vi "OscConnect-Com-Exec.vi"(8 "error in (no error)":errorcluster, 9 "ControlQueue":refnum<queue>, 10 "data":variant, 11 "Oscilloscope in":refnum<class "Oscilloscope.lvclass">) -> (0 "error out":errorcluster, 3 "Oscilloscope out":refnum<class "Oscilloscope.lvclass">)   [LabVIEW 2015, in "Oscilloscope.lvclass"]
uses:
  Oscilloscope.lvclass
  dependecies/ControlsVIs/Clusters-def/SERVER-Commands.ctl
  dependecies/ControlsVIs/Clusters-def/OSc-Reply-to-Connect.ctl
  dependecies/ControlsVIs/Clusters-def/OSc-Reply-Connect-client.ctl
  GeneralFunctionality/GeneralFunctionality.lvclass/GeneralFunctionality.ctl
  Control/Control-Server/Control-Server.lvclass
  GeneralFunctionality/GeneralFunctionality.lvclass
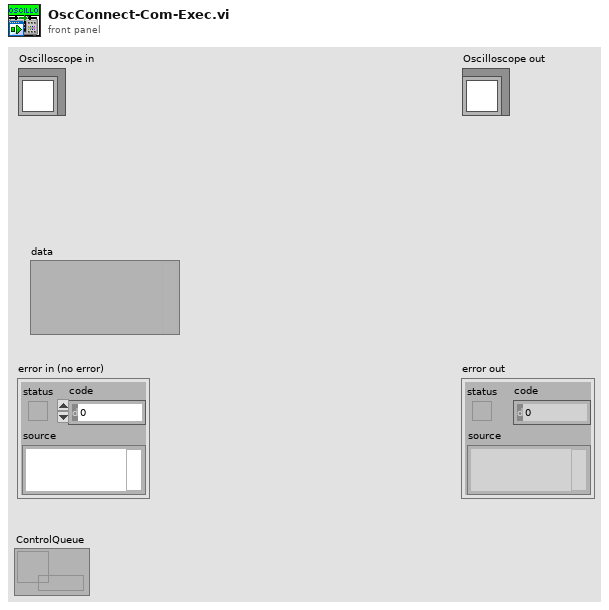
[diagram p1: front panel]
types:
  T1 = typedef "Control-Server.lvclass/SERVER-Commands.ctl" = string
  T2 = typedef "Oscilloscope.lvclass/OSc-Reply-Connect-Client.ctl" = cluster{"on/off":bool, "WCM_state":bool, "error":errorcluster}
  T3 = typedef "Oscilloscope.lvclass/OSc-Reply-to-Connect.ctl" = cluster{"On/Off":bool, "error":errorcluster, "Oscilloscope.lvclass":refnum<class "Oscilloscope.lvclass">}
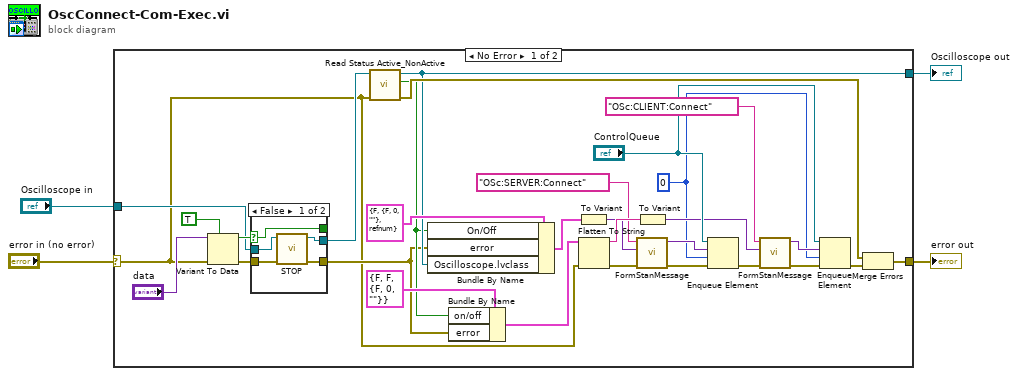
[diagram p0: block diagram]
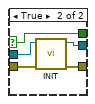
[diagram p2: hidden frame]
diagram:
  n1 = case shown="No Error" "error in (no error)" {
    selector: "error in (no error)" -> [w18 w46]
    tunnel: [w27 w46] -> w3
    tunnel: [w25 w45] -> w1
    tunnel: "Oscilloscope in" -> [w30 w45]
    frame No Error {
      w5 = 0 ("timeout en ms (-1)")
      n2 = Variant To Data(error in=w18, type=TRUE, Variant="data") -> (data=w32:bool, error out=w31:errorcluster)
      n3 = case shown="False" w32 {
        selector: w32 -> [w35 w40]
        tunnel: w31 -> [w39 w44]
        tunnel: w30 -> [w37 w43]
        tunnel: [w36 w42] -> w24
        tunnel: [w38 w41] -> w21
        tunnel: [w35 w40] -> _
        frame False {
          n4 = call-dynamic "STOP.vi"("error in (no error)"=w39, "Stop in"=w37) -> ("error out"=w38:errorcluster, "Stop out"=w36:refnum<class "Oscilloscope.lvclass">)  [unwired: 8 in]
        }
        frame True {
          n5 = call-dynamic "INIT.vi"("error in (no error)"=w44, "GeneralFunctionality in"=w43) -> ("error out"=w41:errorcluster, "GeneralFunctionality out"=w42:refnum<class "Oscilloscope.lvclass">)  [unwired: 8 in]
        }
      }
      n6 = call "Read Status Active_NonActive.vi"("error in (no error)"=w18, "GeneralFunctionality in"=w24) -> ("error out"=w28:errorcluster, "Status Active/NonActive"=w22:bool, "GeneralFunctionality out"=w25:refnum<class "Oscilloscope.lvclass">)  [unwired: 7 in]
      n7 = Bundle By Name(cluster=T3 {"On/Off"=FALSE, "error"={"status"=FALSE, "code"=0, "source"=""}, "Oscilloscope.lvclass"=refnum} ("Cluster"), "On/Off"=w22, "error"=w21, "Oscilloscope.lvclass"=w25) -> (w29:T3)
      n8 = Bundle By Name(cluster=T2 {"on/off"=FALSE, "WCM_state"=FALSE, "error"={"status"=FALSE, "code"=0, "source"=""}} ("output cluster"), "on/off"=w22, "error"=w21) -> (w20:T2)
      n9 = To Variant(anything=w29) -> (Variant=w8:variant)
      n10 = Flatten To String(anything=w20, error in (no error)=w18) -> (data string=w19:string, error out=w16:errorcluster)  [unwired: 2 in, 1 out]
      n11 = call "FormStanMessage.vi"("error in"=w16, "data"=w8, "Command"=T1 "OSc:SERVER:Connect" ("Commands")) -> ("error out"=w15:errorcluster, "message"=w14:variant)  [unwired: 7 in]
      n12 = To Variant(anything=w19) -> (Variant=w6:variant)
      n13 = Enqueue Element(queue="ControlQueue", element=w14, timeout in ms (-1)=w5, error in (no error)=w15) -> (error out=w13:errorcluster)  [unwired: 2 out]
      n14 = call "FormStanMessage.vi"("error in"=w13, "data"=w6, "Command"=T1 "OSc:CLIENT:Connect" ("Commands")) -> ("error out"=w12:errorcluster, "message"=w7:variant)  [unwired: 7 in]
      n15 = Enqueue Element(queue="ControlQueue", element=w7, timeout in ms (-1)=w5, error in (no error)=w12) -> (error out=w11:errorcluster)  [unwired: 2 out]
      n16 = Merge Errors(w28, w11) -> (w27:errorcluster)
    }
    frame Error {
    }
  }
  "error out" <- w3
  "Oscilloscope out" <- w1
